vi "SLM Reset.vi"   [LabVIEW 2022 SP3]
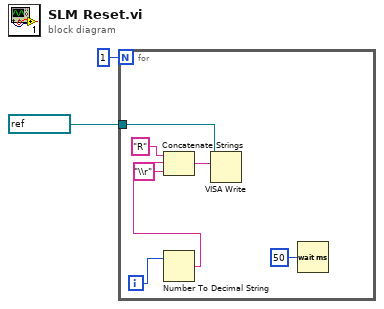
[diagram p0: block diagram]
diagram:
  n1 = for {
    N: 1 -> [_]
    tunnel: refnum<visa-resource-name> "COM9" ("VISA resource name") -> [w9]
    i -> [w8]
    n2 = Number To Decimal String(number=w8) -> (decimal integer string=w6:string)  [unwired: 1 in]
    n3 = Concatenate Strings("R" ("string"), w6, "\\r" ("string")) -> (w4:string)
    n4 = VISA Write(VISA resource name=w9, write buffer=w4) -> ()  [unwired: 1 in, 3 out]
    n5 = Wait (ms)(milliseconds to wait=u32 50) -> ()  [unwired: 1 out]
  }
